vi "Validate Arguments.vi"(8 "error in (no error)":errorcluster, 11 "InitAction in":refnum<class "InitAction.lvclass">) -> (0 "error out":errorcluster, 2 "Problems":string[](array[string]), 3 "InitAction out":refnum<class "InitAction.lvclass">)   [LabVIEW 2020, in "GPackTools.lvlib" / "InitAction.lvclass"]
uses:
  InitAction.lvclass
  InitAction.lvclass/InitAction.ctl
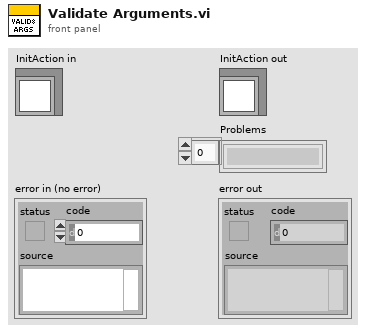
[diagram p1: front panel]
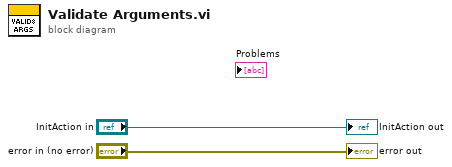
[diagram p0: block diagram]
diagram:
  "error out" <- "error in (no error)"
  "InitAction out" <- "InitAction in"
